vi "attribute_read_string_simple.vi"(5 "Repeated Capability":string, 7 "Attribute":T1={"Identifier"="", "Descriptive name"="", "Data Type"=enum."Integer 32", "Command"="", "Access"=2, "Range Table"="", "Read Callback"="", "Write Callback"="", "Range Callback"="", "Check Callback"="", "Rngtable Callback"="", "Coerce Callback"="", "Supported Models"="", "Instrument Options"="", "Repeated Capabilities"="", "Check Status Callback"="", "Index"=0, "Flag: OPC Wait"=FALSE, "Flag: Dont check status"=FALSE, "Flag: Cache Only"=FALSE} {"Access" items=["Read Only", "Write Only", "Read/Write"]}, 8 "error in":errorcluster, 10 "Direct Attribute ID (\"\")":string, 11 "VISA resource name":refnum<visa-resource-name>) -> (0 "error out":errorcluster, 2 "string out":string, 3 "VISA resource name out":refnum<visa-resource-name>)   [LabVIEW 2014, in "rszvl_rsidr_core.lvlib"]
uses:
  rszvl_rsidr_core.lvlib
  type_Attribute.ctl
  type_Attribute_Data_Type.ctl
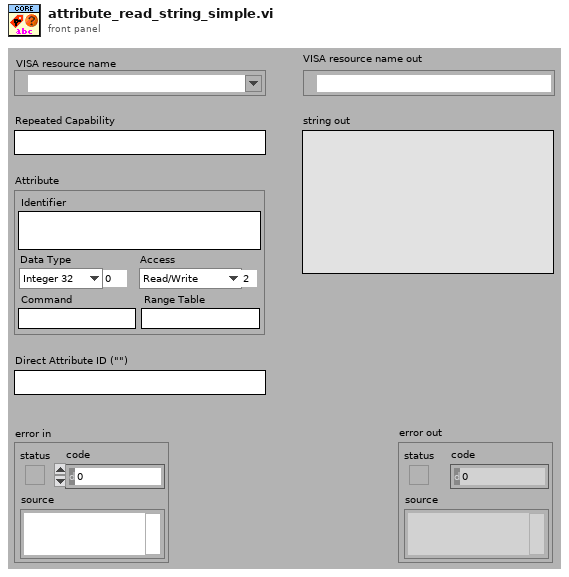
[diagram p1: front panel]
types:
  T1 = typedef "rszvl_rsidr_core.lvlib/type_Attribute.ctl" = cluster{"Identifier":string, "Descriptive name":string, "Data Type":T2, "Command":string, "Access":u16, "Range Table":string, "Read Callback":string, "Write Callback":string, "Range Callback":string, "Check Callback":string, "Rngtable Callback":string, "Coerce Callback":string, "Supported Models":string, "Instrument Options":string, "Repeated Capabilities":string, "Check Status Callback":string, "Index":i32, "Flag: OPC Wait":bool, "Flag: Dont check status":bool, "Flag: Cache Only":bool}
  T2 = typedef "rszvl_rsidr_core.lvlib/type_Attribute_Data_Type.ctl" = enum16{"Integer 32", "Double", "String", "Boolean", "None", "Integer 64"}
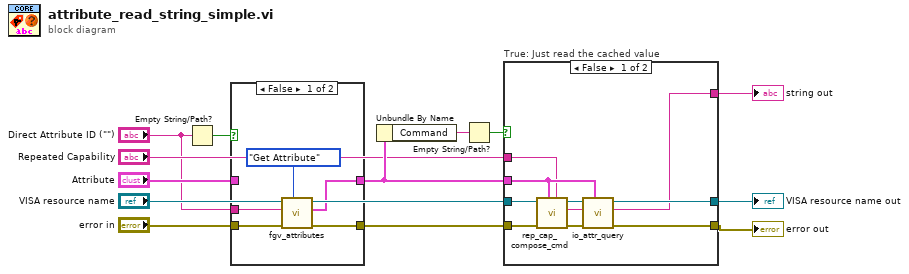
[diagram p0: block diagram]
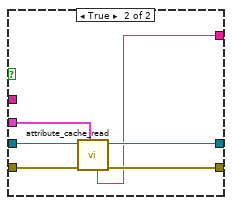
[diagram p3: hidden frame]
diagram:
  n1 = Empty String/Path?(string/path="Direct Attribute ID (\"\")") -> (empty?=w12:bool)
  n2 = case shown="False" w12 {
    tunnel: "error in" -> [w18 w19]
    tunnel: [w17 w19] -> w13
    tunnel: "Direct Attribute ID (\"\")" -> [w16 _]
    tunnel: "Attribute" -> [_ w20]
    tunnel: [w14 w20] -> w11
    frame False {
      n3 = call "fgv_attributes.vi"("Operation"=enum16{"Initialize", "Get Attribute"}."Get Attribute", "error in"=w18, "Attribute ID in"=w16) -> ("error out"=w17:errorcluster, "Attribute out"=w14:T1)  [unwired: 6 in, 1 out]
    }
    frame True {
    }
  }
  n4 = Unbundle By Name(w11) -> ("Command"=w10:string)
  n5 = Empty String/Path?(string/path=w10) -> (empty?=w9:bool)
  n6 = case "True: Just read the cached value" shown="False" w9 {
    tunnel: "Repeated Capability" -> [w22 _]
    tunnel: [w25 w33] -> w1
    tunnel: [w24 w32] -> w2
    tunnel: [w21 w31] -> w3
    tunnel: "VISA resource name" -> [w28 w35]
    tunnel: w13 -> [w29 w36]
    tunnel: w11 -> [w23 w34]
    frame False {
      n7 = call "rep_cap_compose_cmd.vi"("Repeated Capability"=w22, "Attribute"=w23, "error in"=w29, "VISA resource name"=w28) -> ("error out"=w27:errorcluster, "Command out"=w30:string, "VISA resource name out"=w26:refnum<visa-resource-name>)  [unwired: 5 in]
      n8 = call "io_attr_query.vi"("Attribute"=w23, "error in"=w27, "write buffer"=w30, "VISA resource name"=w26) -> ("error out"=w25:errorcluster, "read buffer"=w21:string, "VISA resource name out"=w24:refnum<visa-resource-name>)  [unwired: 5 in]
    }
    frame True {
      n9 = call "attribute_cache_read.vi"("Attribute"=w34, "error in"=w36, "VISA resource name"=w35) -> ("error out"=w33:errorcluster, "VISA resource name out"=w32:refnum<visa-resource-name>, "String out"=w31:string)  [unwired: 1 in, 5 out]
    }
  }
  "error out" <- w1
  "VISA resource name out" <- w2
  "string out" <- w3
